vi "Confirmation Dialog.vi"(4 "Middle Button Visible?":bool, 5 "Window Title (\"\")":string, 6 "Calling VI in":refnum<vi>, 7 "Message":string, 8 "error in (no error)":errorcluster, 9 "Right Button Text (\"Cancel\")":string="Cancel", 10 "Middle Button Text (\"No\")":string="No", 11 "Left Button Text (\"OK\")":string="OK") -> (0 "error out":errorcluster, 2 "Skip Prompts?":bool, 3 "Which Button?":T1(ring)=enum."Center Button")   [LabVIEW 2020, in "VI Properties Editor.lvlib"]
doc: "Displays a generic confirmation dialog with various options."
uses:
  VI Properties Editor.lvlib
panel:
  in  "Middle Button":bool
  out "Message Display":string
  in  "Skip Prompts":bool caption="Don't show this dialog again (you can\nreactivate this dialog in Options later)"
  in  "Right Button":bool
  in  "Left Button":bool
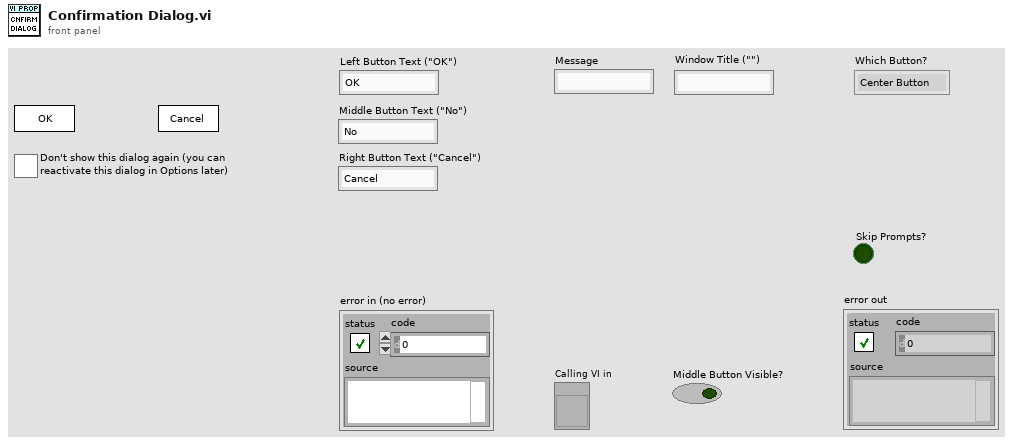
[diagram p1: front panel]
types:
  T1 = enum16{"Left Button", "Center Button", "Right Button", "Window Close"}
  T2 = enum32{"Invalid", "Standard", "Closed", "Hidden", "Minimized", "Maximized"}
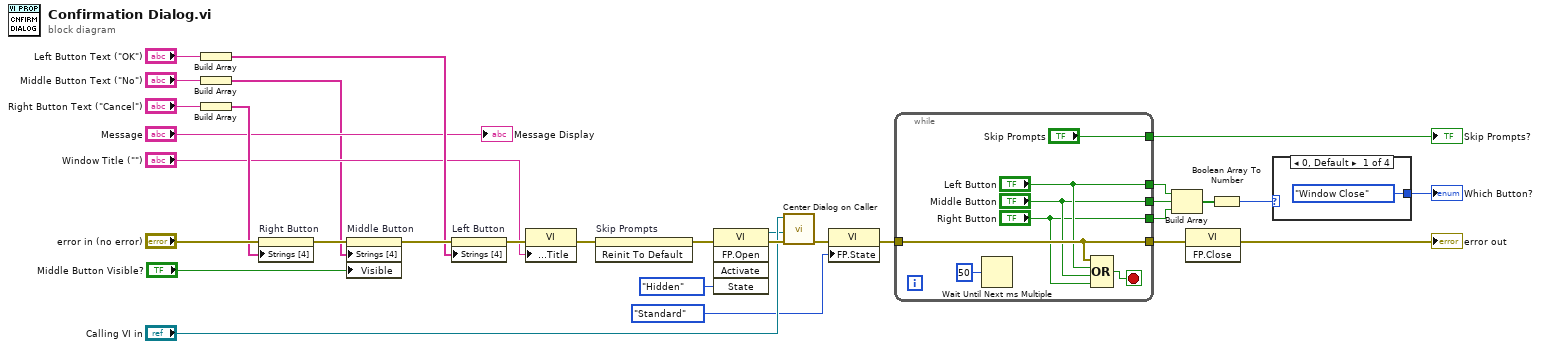
[diagram p0: block diagram]
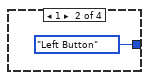
[diagram p2: hidden frame]
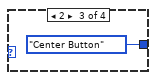
[diagram p3: hidden frame]
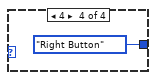
[diagram p4: hidden frame]
diagram:
  n1 = Build Array("Left Button Text (\"OK\")") -> (w21:string[])
  n2 = Build Array("Middle Button Text (\"No\")") -> (w5:string[])
  n3 = Build Array("Right Button Text (\"Cancel\")") -> (w23:string[])
  n4 = property on="Right Button" class="Bool"(error in="error in (no error)", "Strings [4]"=w23) -> (error out=w25:errorcluster)  [unwired: 1 in, 1 out]
  n5 = property on="Middle Button" class="Bool"(error in=w25, "Strings [4]"=w5, "Visible"="Middle Button Visible?") -> (error out=w24:errorcluster)  [unwired: 1 in, 1 out]
  n6 = property on="Left Button" class="Bool"(error in=w24, "Strings [4]"=w21) -> (error out=w28:errorcluster)  [unwired: 1 in, 1 out]
  n7 = property class="VI"(error in=w28, "Front Panel.Title"="Window Title (\"\")") -> (error out=w3:errorcluster)  [unwired: 1 in, 1 out]
  n8 = invoke on="Skip Prompts" class="Bool (strict)" method="Reinit To Default"(error in=w3) -> (error out=w2:errorcluster)  [unwired: 2 in, 2 out]
  n9 = invoke class="VI" method="FP.Open"(error in=w2, "State"=T2."Hidden") -> (reference out=w14:refnum<vi>, error out=w26:errorcluster)  [unwired: 3 in, 3 out]
  n10 = call "Center Dialog on Caller.vi"("error in (no error)"=w26, "Dialog VI"=w14, "Calling VI in"="Calling VI in") -> ("error out"=w27:errorcluster)  [unwired: 7 in, 1 out]
  n11 = property class="VI"(error in=w27, "FP.State"=T2."Standard" ("Front Panel Window:State")) -> (error out=w1:errorcluster)  [unwired: 1 in, 1 out]
  n12 = while {
    tunnel: w1 -> [w38]
    tunnel: [w38] -> w30
    tunnel: ["Skip Prompts"] -> w19
    tunnel: ["Left Button"] -> w12
    tunnel: ["Middle Button"] -> w11
    tunnel: ["Right Button"] -> w10
    stop <- w36 stop-if-true
    n13 = Wait Until Next ms Multiple(millisecond multiple=u32 50) -> ()  [unwired: 1 out]
    n14 = Compound Arithmetic op=OR(w38, "Left Button", "Middle Button", "Right Button") -> (w36:bool)
  }
  "Skip Prompts?" <- w19
  n15 = Build Array(w12, w11, w10) -> (w9:bool[])
  n16 = invoke class="VI" method="FP.Close"(error in=w30) -> (error out=→"error out":errorcluster)  [unwired: 2 in, 2 out]
  n17 = Boolean Array To Number(Boolean array=w9) -> (number=w8:u32)
  n18 = case shown="0, Default" w8 {
    tunnel: [T1."Window Close" ("Which Button?") T1."Left Button" ("Which Button?") T1."Center Button" ("Which Button?") T1."Right Button" ("Which Button?")] -> w7
    frame 0, Default {
    }
    frame 1 {
    }
    frame 2 {
    }
    frame 4 {
    }
  }
  "Which Button?" <- w7
  "Message Display" <- "Message"
